vi "channel operation tests.vi"() -> ()   [LabVIEW 2013, in "Shared Library Module tests.lvlib"]
doc: "Platypus Framework 1.0.1.60\nNI Systems Engineering - National Instruments"
uses:
  Shared Library Module tests.lvlib
  <vilib>/NI/Tag Bus Module Framework/channel/channel classification.ctl
  configuration/Shared Library Module configuration.lvclass
  <vilib>/NI/Tag Bus Module Framework/channel/TBM channel.lvclass
  <vilib>/NI/Tag Bus Module Framework/root configuration/TBM configuration.lvclass
panel:
  out "channels match":bool
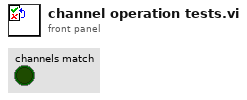
[diagram p1: front panel]
types:
  T1 = typedef "TBM channel.lvclass/channel classification.ctl" = enum16{"input data", "output data", "processing parameter", "processing result"}
  T2 = typedef "tag bus.lvlib/tag descriptor.lvclass/Data Type.ctl" = enum16{"Double", "Single", "I64", "I32", "I16", "I8", "U64", "U32", "U16", "U8", "Boolean", "String", "Array of Double", "Array of Single", "Array of I64", "Array of I32", "Array of I16", "Array of I8", "Array of U64", "Array of U32", "Array of U16", "Array of U8", "Array of Boolean", "Array of String"}
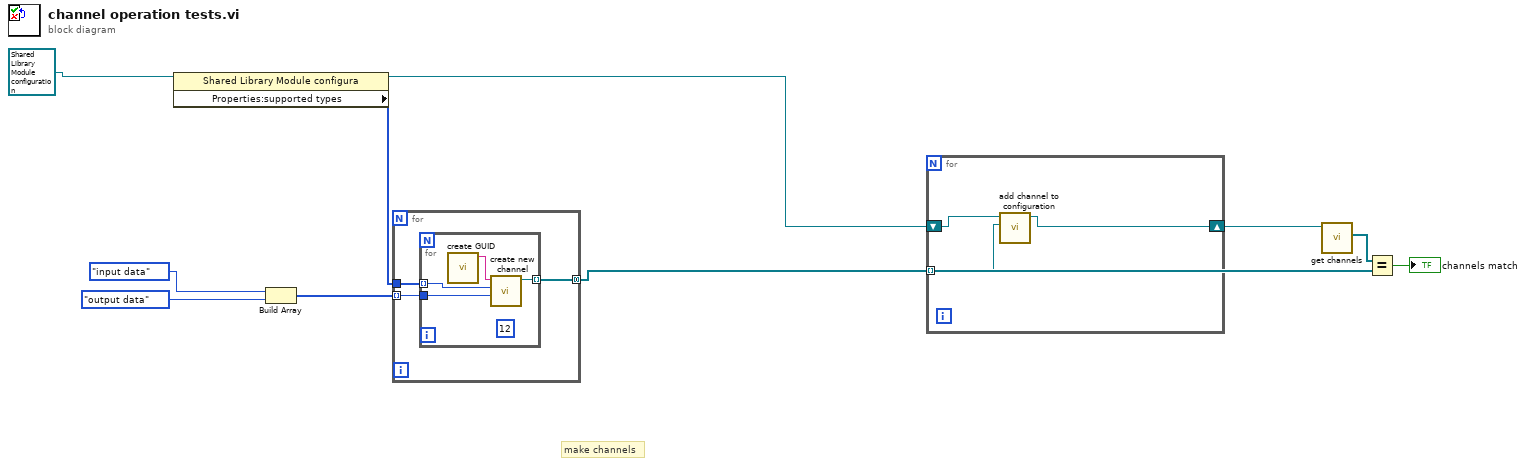
[diagram p0: block diagram]
diagram:
  # "make channels"
  n1 = property class="Shared Library Module configura"(reference=refnum<class "Shared Library Module configuration.lvclass"> refnum ("tag bus configurable plugin module configuration")) -> (reference out=w2:refnum<class "Shared Library Module configuration.lvclass">, "Properties:supported types"=w7:T2[])  [unwired: 1 in, 1 out]
  n2 = Build Array(channel_classification."input data" ("channel classification"), channel_classification."output data" ("channel classification")) -> (w8:T1[])
  n3 = for {
    tunnel: w8 -> [w13] mode=indexing
    tunnel: [w11] -> w3 mode=concatenating
    tunnel: w7 -> [w12]
    n4 = for {
      tunnel: w13 -> [w16]
      tunnel: [w17] -> w11 mode=indexing
      tunnel: w12 -> [w15] mode=indexing
      (unwired) 12
      n5 = call <vilib>:"create GUID.vi"() -> ("uuid"=w14:string)  [unwired: 11 in]
      n6 = call <vilib>:"create new channel.vi"("channel classification"=w16, "data type"=w15, "channel name"=w14) -> ("channel"=w17:refnum<class "TBM channel.lvclass">)  [unwired: 8 in]
    }
  }
  n7 = for {
    tunnel: w3 -> [w18] mode=indexing
    shift-right: [w19] -> w1
    shift-left: w2 -> [w20]
    n8 = call "add channel to configuration.vi"("TBM channel in"=w18, "Shared Library Module configuration in"=w20) -> ("Shared Library Module configuration out"=w19:refnum<class "Shared Library Module configuration.lvclass">)  [unwired: 8 in, 1 out]
  }
  n9 = call-dynamic "get channels.vi"("Shared Library Module configuration in"=w1) -> ("channels"=w6:refnum<class "TBM channel.lvclass">[])  [unwired: 9 in, 1 out]
  n10 = Equal?(x=w6, y=w3) -> (x = y?=→"channels match":bool)
